vi "Module State.vi"(10 "Modules In":T1[](array[typedef]), 11 "Data In":u16[](array[numeric])) -> (2 "Modules Out":T1[](array[typedef]), 3 "Board Out":T1)   [LabVIEW 2018, in "Control Box.lvlib" / "Control Box.lvclass"]
uses:
  Control Box.lvclass
  Custom Controls/Channel Status.ctl
  Control Box.lvlib
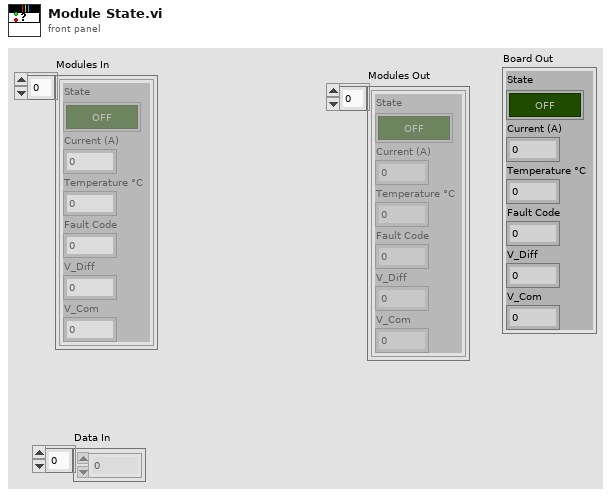
[diagram p1: front panel]
types:
  T1 = typedef "Control Box.lvlib/Channel Status.ctl" = cluster{"State":bool, "Current (A)":dbl, "Temperature °C":dbl, "Fault Code":u8, "V_Diff":dbl, "V_Com":dbl}
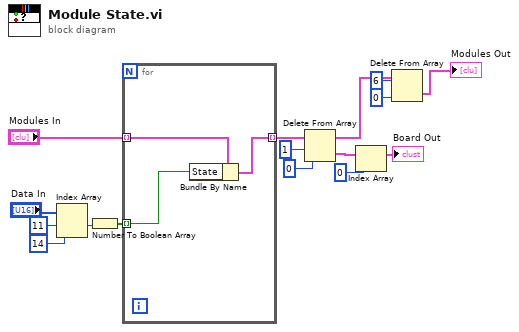
[diagram p0: block diagram]
diagram:
  n1 = Index Array(array="Data In", index #1=11 ("index"), index #2=14 ("index")) -> (element #1=w12:u16)  [unwired: 1 out]
  n2 = Number To Boolean Array(number=w12) -> (Boolean array=w11:bool[])
  n3 = for {
    tunnel: "Modules In" -> [w19] mode=indexing
    tunnel: w11 -> [w18] mode=indexing
    tunnel: [w17] -> w10 mode=indexing
    n4 = Bundle By Name(cluster=w19, "State"=w18) -> (w17:T1)
  }
  n5 = Delete From Array(array=w10, length=1, index=0) -> (deleted portion=w8:T1[], array with subset deleted=w4:T1[])
  n6 = Index Array(array=w8, index=0) -> (element=→"Board Out":T1)
  n7 = Delete From Array(array=w4, length=6, index=0) -> (deleted portion=→"Modules Out":T1[])  [unwired: 1 out]
